vi "Computer Sequence Simulation Dialog.vi"(4 "Sequence Context":T1) -> (0 "error out":errorcluster, 1 "Test Data":T2 {"Numeric Measurement" format="%.2f"})   [LabVIEW 2010]
uses:
  <vilib>/addons/TestStand/_TSLegacy.llb/LabVIEW Test - Test Data.ctl
  <vilib>/addons/TestStand/_TSLegacy.llb/LabVIEW Test - Sequence Context.ctl
panel:
  in  "CPU":bool
  in  "OK":bool
  in  "Keyboard":bool
  in  "RAM":bool
  in  "ROM":bool
  in  "Video":bool
  in  "Power":bool=TRUE
  # "Check tests that should fail:"
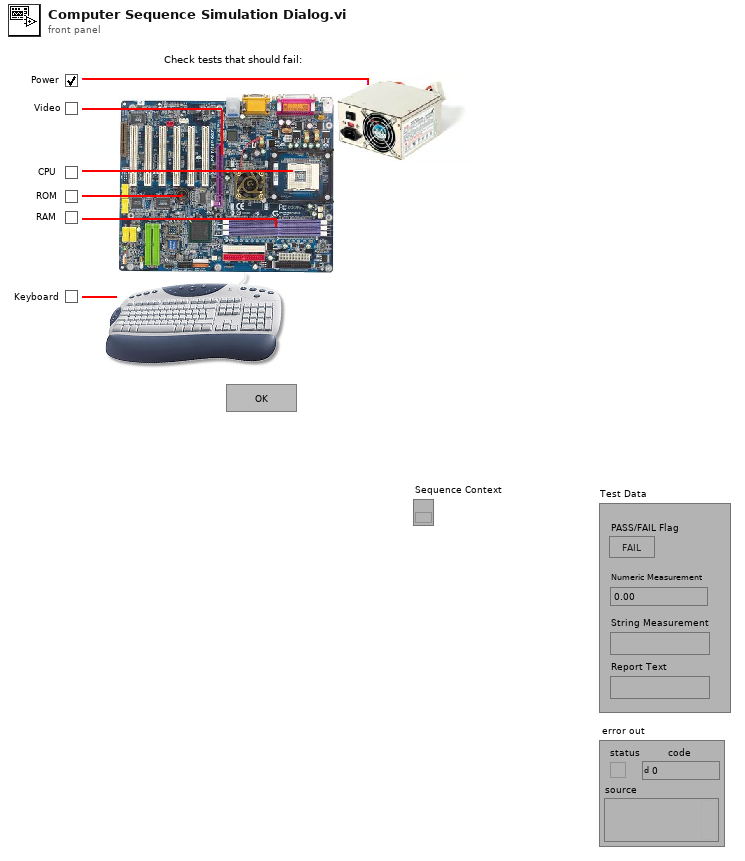
[diagram p1: front panel]
types:
  T1 = typedef "LabVIEW Test - Sequence Context.ctl" = refnum<k7>
  T2 = typedef "LabVIEW Test - Test Data.ctl" = cluster{"PASS/FAIL Flag":bool, "Numeric Measurement":dbl, "String Measurement":string, "Report Text":string}
  T3 = typedef "TestStand - Status Monitor.ctl" = cluster{"Execution":refnum<k7>, "Termination Monitor":refnum<k7>, "Sequence Context":refnum<k7>}
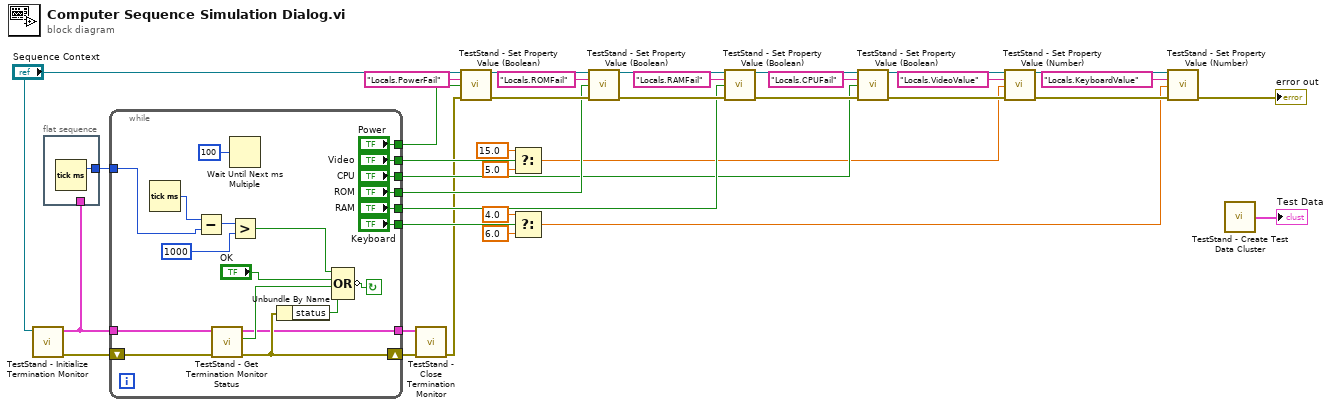
[diagram p0: block diagram]
diagram:
  n1 = call "TestStand - Initialize Termination Monitor.vi"("Sequence Context In"="Sequence Context") -> ("error out"=w6:errorcluster, "Status Monitor Out"=w2:T3)  [unwired: 1 in, 8 out]
  n2 = flat-sequence {
    tunnel: [w38] -> w1
    tunnel: w2 -> [_]
    frame #0 {
      n3 = Tick Count (ms)() -> (millisecond timer value=w38:u32)
    }
  }
  n4 = while {
    tunnel: w2 -> [w44]
    tunnel: [w45] -> w3
    shift-left: w6 -> [w49]
    shift-right: [w46] -> w5
    tunnel: ["Keyboard"] -> w34
    tunnel: ["RAM"] -> w22
    tunnel: ["ROM"] -> w26
    tunnel: ["CPU"] -> w18
    tunnel: ["Video"] -> w37
    tunnel: ["Power"] -> w30
    tunnel: w1 -> [w40]
    stop <- w51 continue-if-true
    n5 = Tick Count (ms)() -> (millisecond timer value=w42:u32)
    n6 = Subtract(x=w42, y=w40) -> (x-y=w41:u32)
    n7 = call "TestStand - Get Termination Monitor Status.vi"("error in (no error)"=w49, "Status Monitor In"=w44) -> ("error out"=w46:errorcluster, "Terminating or Aborting"=w48:bool, "Status Monitor Out"=w45:T3)  [unwired: 7 out]
    n8 = Wait Until Next ms Multiple(millisecond multiple=u32 100) -> ()  [unwired: 1 out]
    n9 = Greater?(x=w41, y=u32 1000) -> (0:w39:bool)
    n10 = Unbundle By Name(w46) -> ("status"=w47:bool)
    n11 = Compound Arithmetic op=OR(w39, "OK", w48, w47) -> (invert w51:bool)
  }
  n12 = call "TestStand - Close Termination Monitor.vi"("error in (no error)"=w5, "Status Monitor In"=w3) -> ("error out"=w4:errorcluster)  [unwired: 9 out]
  n13 = call <vilib>:"TestStand - Set Property Value (Boolean).vi"("Sequence Context In"="Sequence Context", "Lookup String"="Locals.PowerFail" ("lookupString"), "New Value"=w30, "error in (no error)"=w4) -> ("Sequence Context Out"=w29:refnum<k7>, "error out"=w28:errorcluster)  [unwired: 1 in, 9 out]
  n14 = Select(t=15.0, s=w37, f=5.0) -> (s? t:f=w14:dbl)
  n15 = Select(t=4.0, s=w34, f=6.0) -> (s? t:f=w10:dbl)
  n16 = call <vilib>:"TestStand - Set Property Value (Boolean).vi"("Sequence Context In"=w29, "Lookup String"="Locals.ROMFail" ("lookupString"), "New Value"=w26, "error in (no error)"=w28) -> ("Sequence Context Out"=w23:refnum<k7>, "error out"=w24:errorcluster)  [unwired: 1 in, 9 out]
  n17 = call <vilib>:"TestStand - Set Property Value (Boolean).vi"("Sequence Context In"=w23, "Lookup String"="Locals.RAMFail" ("lookupString"), "New Value"=w22, "error in (no error)"=w24) -> ("Sequence Context Out"=w19:refnum<k7>, "error out"=w20:errorcluster)  [unwired: 1 in, 9 out]
  n18 = call <vilib>:"TestStand - Set Property Value (Boolean).vi"("Sequence Context In"=w19, "Lookup String"="Locals.CPUFail" ("lookupString"), "New Value"=w18, "error in (no error)"=w20) -> ("Sequence Context Out"=w16:refnum<k7>, "error out"=w17:errorcluster)  [unwired: 1 in, 9 out]
  n19 = call <vilib>:"TestStand - Set Property Value (Number).vi"("Sequence Context In"=w16, "Lookup String"="Locals.VideoValue" ("lookupString"), "New Value"=w14, "error in (no error)"=w17) -> ("Sequence Context Out"=w11:refnum<k7>, "error out"=w12:errorcluster)  [unwired: 1 in, 9 out]
  n20 = call <vilib>:"TestStand - Set Property Value (Number).vi"("Sequence Context In"=w11, "Lookup String"="Locals.KeyboardValue" ("lookupString"), "New Value"=w10, "error in (no error)"=w12) -> ("error out"=→"error out":errorcluster)  [unwired: 1 in, 10 out]
  n21 = call "TestStand - Create Test Data Cluster.vi"() -> ("Test Data"=→"Test Data":T2)  [unwired: 4 in]
